vi "Compile Shared Resources.vi"(8 "error in":errorcluster, 10 "shared resources":refnum<class "Shared Resources.lvclass">, 11 "device ref in":T1=18446744073709551615 format="%.0x") -> (0 "error out":errorcluster, 2 "flattened shared resources":string, 3 "device ref out":T1=18446744073709551615 format="%.0x")   [LabVIEW 2020, in "AIM MIL-STD-1553 System Explorer.lvlib"]
uses:
  AIM MIL-STD-1553 System Explorer.lvlib
  <vilib>/NI VeriStand/Custom Device API/Custom Device Item Ref.ctl
  Includes/AIM MIL-STD-1553 Engine.lvlibp/Engine/Interfaces/Shared Resources/Shared Resources.lvclass
  <vilib>/NI VeriStand/Custom Device API/Custom Device API.lvlib
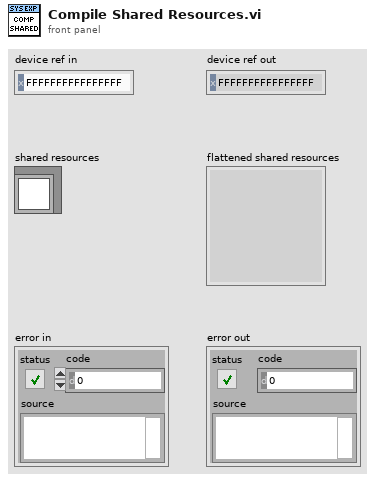
[diagram p1: front panel]
types:
  T1 = typedef "Custom Device API.lvlib/Custom Device Item Ref.ctl" = u64
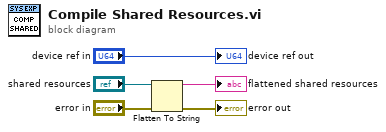
[diagram p0: block diagram]
diagram:
  n1 = Flatten To String(anything="shared resources", error in (no error)="error in") -> (data string=→"flattened shared resources":string, error out=→"error out":errorcluster)  [unwired: 2 in, 1 out]
  "device ref out" <- "device ref in"
